vi "Has Disconnected.vi"(8 "error in (no error)":errorcluster, 11 "Session in":refnum<class "Session.lvclass">) -> (0 "error out":errorcluster, 2 "has disconnected?":bool, 3 "Session out":refnum<class "Session.lvclass">)   [LabVIEW 2020, in "NI_SFTP.lvlib" / "Session.lvclass"]
uses:
  <vilib>/net/SFTP/Session/Session.lvclass
  <vilib>/net/SFTP/Session/Session.lvclass/Session.ctl
  <vilib>/net/SFTP/Low Level Connection/Low Level Connection.lvclass
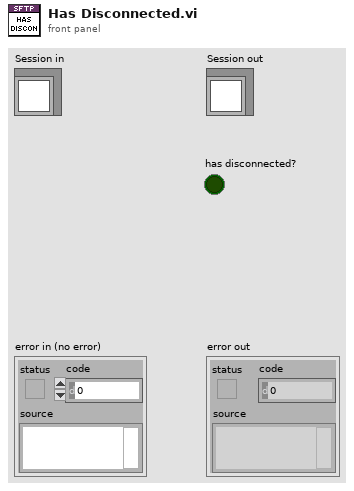
[diagram p1: front panel]
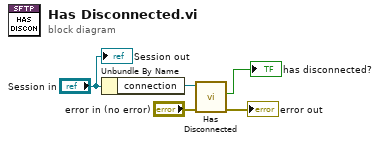
[diagram p0: block diagram]
diagram:
  n1 = Unbundle By Name("Session in") -> ("connection"=w4:refnum<class "Low Level Connection.lvclass">)
  n2 = call <vilib>:"Has Disconnected.vi"("error in (no error)"="error in (no error)", "Low Level Connection in"=w4) -> ("error out"=→"error out":errorcluster, "has disconnected?"=→"has disconnected?":bool)  [unwired: 7 in, 1 out]
  "Session out" <- "Session in"
